vi "svx_DAQ_MaxOrderRead.vi"(4 "error in (no error)":errorcluster, 6 "Container State":T11, 7 "Display State In":T1={"Channel Info Array"=[], "Timing Mode"=enum."Time", "Timing Control 1"=25600.0, "Timing Control 2"=2560.0, "Timing Control 3"=16, "Timing Indicator 1"=0.1, "Reference Visible?"=FALSE, "Reference Type"=enum."<none>", "Tachometer Channel"="", "Tach Pulses Per Rev"=1, "Tach Direction"=enum."CW", "Tach Slope"=enum."Rising", "Tach Threshold"=0.0, "Trigger Channel"="", "Trigger Level"=20.0, "Pretrigger Samples"=1, "Trigger Slope"=enum."Falling", "Trigger Hysteresis"=0.0, "Logging Visible?"=FALSE, "Enable Logging"=FALSE, "Logfile Path"=path "c:/test.tdms"} {"Timing Control 2" format="%#_6f"; "Channel Info Array"."Max" min=0.0 format="± %^#_4g"; "Channel Info Array"."Channel Type" items=["Voltage (V)"=0, "Charge (C)"=9, "-"=99, "SPL (Pa)"=3, "Force (lbf)"=6, "Force (N)"=1, "Acceleration (g) - IEPE"=2, "Acceleration (g) - Charge"=12, "Acceleration (g) - 4 wire DC Voltage"=22, "Velocity (in/s)"=7, "Velocity (mm/s)"=8, "Prox Probe (mil)"=4, "Prox Probe (mm)"=5]}) -> (0 "error out":errorcluster, 2 "Value":i32, 3 "Display State Out":T1={"Channel Info Array"=[], "Timing Mode"=enum."Time", "Timing Control 1"=25600.0, "Timing Control 2"=2560.0, "Timing Control 3"=16, "Timing Indicator 1"=0.1, "Reference Visible?"=FALSE, "Reference Type"=enum."<none>", "Tachometer Channel"="", "Tach Pulses Per Rev"=1, "Tach Direction"=enum."CW", "Tach Slope"=enum."Rising", "Tach Threshold"=0.0, "Trigger Channel"="", "Trigger Level"=20.0, "Pretrigger Samples"=1, "Trigger Slope"=enum."Falling", "Trigger Hysteresis"=0.0, "Logging Visible?"=FALSE, "Enable Logging"=FALSE, "Logfile Path"=path "c:/test.tdms"} {"Timing Control 2" format="%#_6f"; "Channel Info Array"."Max" min=0.0 format="± %^#_4g"; "Channel Info Array"."Channel Type" items=["Voltage (V)"=0, "Charge (C)"=9, "-"=99, "SPL (Pa)"=3, "Force (lbf)"=6, "Force (N)"=1, "Acceleration (g) - IEPE"=2, "Acceleration (g) - Charge"=12, "Acceleration (g) - 4 wire DC Voltage"=22, "Velocity (in/s)"=7, "Velocity (mm/s)"=8, "Prox Probe (mil)"=4, "Prox Probe (mm)"=5]})   [LabVIEW 2017, in "SVX NI-DAQmx AI Configuration XControl.xctl"]
uses:
  <vilib>/addons/Sound and Vibration/svt_DAQmx/Configuration XControl/SVX NI-DAQmx AI Configuration XControl.xctl
  <vilib>/_xctls/Container State.ctl
  <vilib>/addons/Sound and Vibration/svt_DAQmx/Configuration XControl/SubVIs/svx_DAQ_State.ctl
  <vilib>/addons/Sound and Vibration/svt_DAQmx/Configuration XControl/Controls/svx_DAQ_ChannelInfo.ctl
  <vilib>/addons/Sound and Vibration/svt_DAQmx/Configuration XControl/Controls/svx_DAQ_ChannelType.ctl
  <vilib>/addons/Sound and Vibration/svt_DAQmx/Configuration XControl/Controls/svx_DAQ_Coupling.ctl
  <vilib>/addons/Sound and Vibration/svt_DAQmx/Configuration XControl/Controls/svx_DAQ_Excitation.ctl
  <vilib>/addons/Sound and Vibration/svt_DAQmx/Configuration XControl/Controls/svx_DAQ_TimingType.ctl
  <vilib>/addons/Sound and Vibration/svt_DAQmx/Configuration XControl/Controls/svx_DAQ_ReferenceType.ctl
  <vilib>/addons/Sound and Vibration/svt_DAQmx/Configuration XControl/Controls/svx_DAQ_RotationDirection.ctl
  <vilib>/addons/Sound and Vibration/svt_DAQmx/Configuration XControl/Controls/svx_DAQ_Tach_Slope.ctl
  <vilib>/addons/Sound and Vibration/svt_DAQmx/Configuration XControl/Controls/svx_DAQ_Trigger_Slope.ctl
  <vilib>/_xctls/XControlSupport.lvlib
panel:
  # "Replace the Value Indicator below with an Indicator of desired type.\nDo not remove this Indicator or the others from the connector pane. \nDo not change the connector pane pattern.\nThe Value Indicator should always be the second terminal from top on the output side in the connector pane."
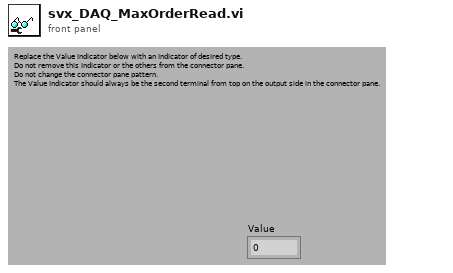
[diagram p1: front panel]
types:
  T1 = typedef "SVX NI-DAQmx AI Configuration XControl.xctl/svx_DAQ_State.ctl" = cluster{"Channel Info Array":T2[], "Timing Mode":T6, "Timing Control 1":dbl, "Timing Control 2":dbl, "Timing Control 3":i32, "Timing Indicator 1":dbl, "Reference Visible?":bool, "Reference Type":T7, "Tachometer Channel":string, "Tach Pulses Per Rev":i32, "Tach Direction":T8, "Tach Slope":T9, "Tach Threshold":dbl, "Trigger Channel":string, "Trigger Level":dbl, "Pretrigger Samples":i32, "Trigger Slope":T10, "Trigger Hysteresis":dbl, "Logging Visible?":bool, "Enable Logging":bool, "Logfile Path":path}
  T2 = typedef "SVX NI-DAQmx AI Configuration XControl.xctl/svx_DAQ_ChannelInfo.ctl" = cluster{"Initialized?":bool, "DAQmx Channel":tag, "Channel Type":T3, "Max":dbl, "Sensitivity":dbl, "Excitation":bool, "Coupling":T4, "Location":string, "Orientation":string, "excitation":T5}
  T3 = typedef "SVX NI-DAQmx AI Configuration XControl.xctl/svx_DAQ_ChannelType.ctl" = u16
  T4 = typedef "SVX NI-DAQmx AI Configuration XControl.xctl/svx_DAQ_Coupling.ctl" = enum16{"AC", "DC"}
  T5 = typedef "svx_DAQ_Excitation.ctl" = enum16{"Off", "Min", "Max"}
  T6 = typedef "SVX NI-DAQmx AI Configuration XControl.xctl/svx_DAQ_TimingType.ctl" = enum16{"Time", "Frequency", "Order"}
  T7 = typedef "SVX NI-DAQmx AI Configuration XControl.xctl/svx_DAQ_ReferenceType.ctl" = enum16{"<none>", "Analog Tachometer", "Analog SW Trigger"}
  T8 = typedef "SVX NI-DAQmx AI Configuration XControl.xctl/svx_DAQ_RotationDirection.ctl" = enum16{"CW", "CCW"}
  T9 = typedef "SVX NI-DAQmx AI Configuration XControl.xctl/svx_DAQ_Tach_Slope.ctl" = enum16{"Rising", "Falling"}
  T10 = typedef "SVX NI-DAQmx AI Configuration XControl.xctl/svx_DAQ_Trigger_Slope.ctl" = enum16{"Falling", "Rising"}
  T11 = typedef "XControlSupport.lvlib/Container State.ctl" = cluster{"Indicator?":bool, "Run Mode?":bool, " Refnum":refnum<vi>}
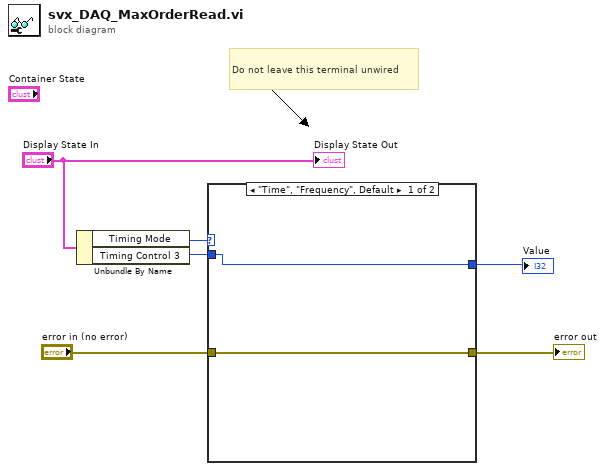
[diagram p0: block diagram]
diagram:
  # "Do not leave this terminal unwired"
  n1 = Unbundle By Name("Display State In") -> ("Timing Mode"=w5:T6, "Timing Control 3"=w4:i32)
  n2 = case shown="\"Time\", \"Frequency\", Default" w5 {
    tunnel: w4 -> [w8 w10]
    tunnel: [w8 w10] -> w3
    tunnel: [w7 w9] -> w2
    tunnel: "error in (no error)" -> [w7 w9]
    frame "Time", "Frequency", Default {
    }
    frame "Order" {
    }
  }
  "error out" <- w2
  "Value" <- w3
  "Display State Out" <- "Display State In"
